vi "Lock Topic.vi"(6 "PublicationPolicy":refnum<class "IPublicationPolicy.lvclass">, 8 "error in (no error)":errorcluster, 9 "Return Error Transport":refnum<class "ITransport.lvclass">, 10 "Publisher ID":string, 11 "Topic in":refnum<class "Topic.lvclass">) -> (0 "error out":errorcluster, 3 "Topic out":refnum<class "Topic.lvclass">)   [LabVIEW 2017, in "Mediator.lvlib" / "Topic.lvclass"]
doc: "<License>\nCopyright © 2017 Composed Systems, LLC | All rights reserved\nwww.composed.io\n\nAuthor: Ethan Stern <ethan.stern@composed.io>\n\nThis software is provided \"AS IS\" WITHOUT WARRANTIES, either express or implied, AND IS FOR EDUCATIONAL PURPOSES ONLY.\n</License>"
uses:
  <vilib>/gpm_packages/@cs/mva-core/Source/Mediator/Topic/Topic.lvclass
  <vilib>/gpm_packages/@cs/transport/Source/ITransport/ITransport.lvclass
  <vilib>/gpm_packages/@cs/mva-core/Source/IMediator/IPublicationPolicy/IPublicationPolicy.lvclass
  <vilib>/gpm_packages/@cs/mva-core/Source/Mediator/Topic/Topic.lvclass/Topic.ctl
  <vilib>/ErrorRing/Error Ring.xnode
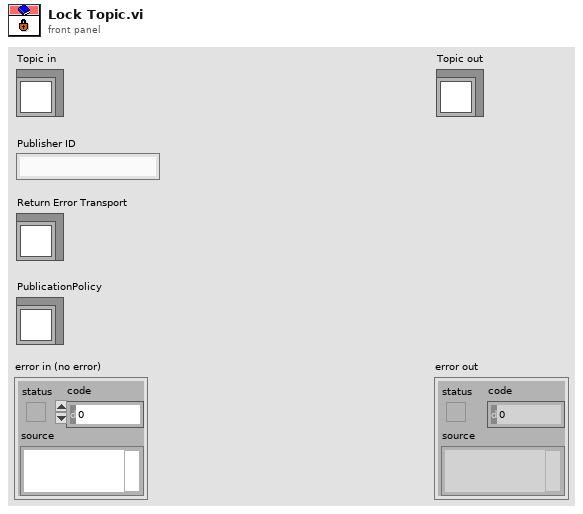
[diagram p1: front panel]
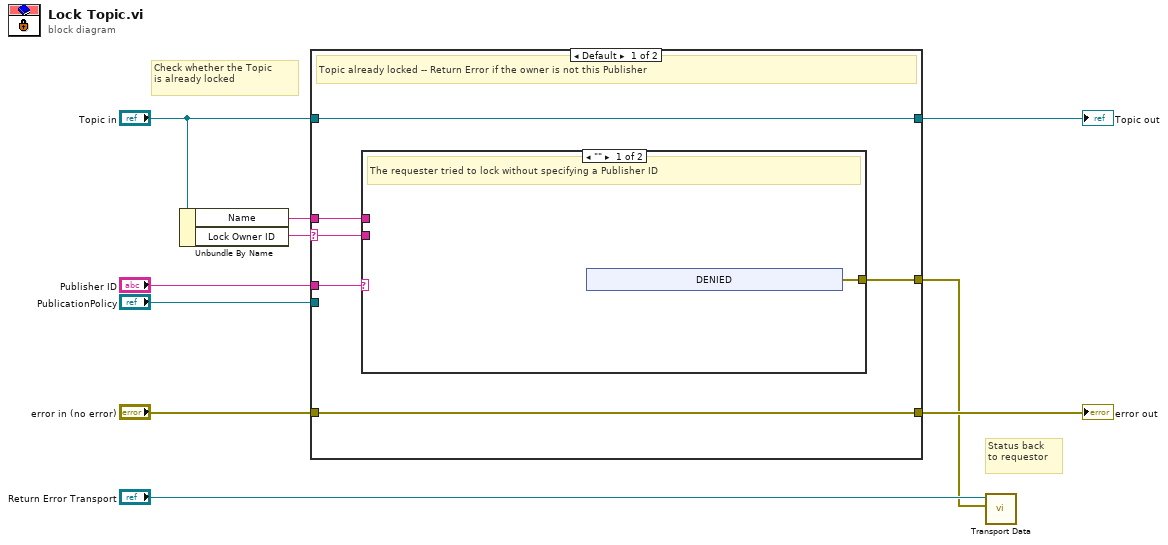
[diagram p0: block diagram]
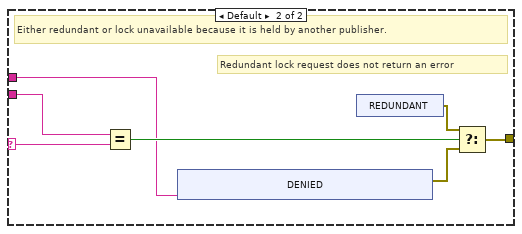
[diagram p2: hidden frame]
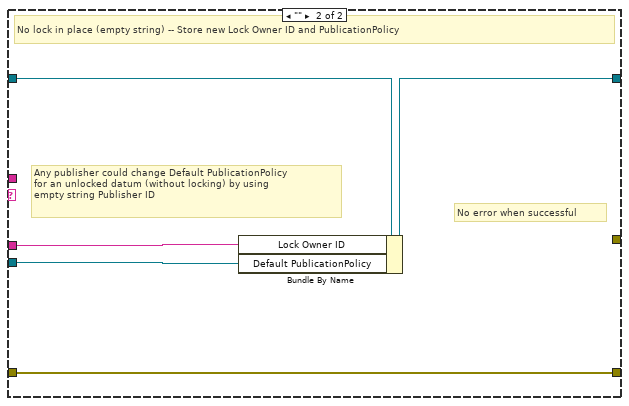
[diagram p3: hidden frame]
diagram:
  # "Status back\nto requestor"
  # "Check whether the Topic\nis already locked"
  n1 = Unbundle By Name("Topic in") -> ("Name"=w1:string, "Lock Owner ID"=w4:string)
  n2 = case shown="Default" w4 {
    selector: w4 -> [w15 _]
    tunnel: "error in (no error)" -> [w16 w33]
    tunnel: [w16 w33] -> w9
    tunnel: [w13 w35] -> w8
    tunnel: "Topic in" -> [w13 w36]
    tunnel: "Publisher ID" -> [w14 w34]
    tunnel: "PublicationPolicy" -> [_ w32]
    tunnel: [w12 _] -> w2
    tunnel: w1 -> [w11 _]
    frame Default {
      # "Topic already locked -- Return Error if the owner is not this Publisher"
      n3 = case shown="\"\"" w14 {
        selector: w14 -> [_ w24]
        tunnel: w15 -> [_ w25]
        tunnel: [w17 w20] -> w12
        tunnel: w11 -> [_ w19]
        frame "" {
          # "The requester tried to lock without specifying a Publisher ID"
          n4 = xnode "DENIED"() -> ("error out"=w17:errorcluster)
        }
        frame Default {
          # "Redundant lock request does not return an error"
          # "Either redundant or lock unavailable because it is held by another publisher."
          n5 = Equal?(x=w25, y=w24) -> (x = y?=w23:bool)
          n6 = xnode "DENIED"("parameter 0"=w19) -> ("error out"=w21:errorcluster)
          n7 = xnode "REDUNDANT"() -> ("error out"=w22:errorcluster)
          n8 = Select(t=w22, s=w23, f=w21) -> (s? t:f=w20:errorcluster)
        }
      }
    }
    frame "" {
      # "No error when successful"
      # "Any publisher could change Default PublicationPolicy\nfor an unlocked datum (without locking) by using\nempty string Publisher ID"
      # "No lock in place (empty string) -- Store new Lock Owner ID and PublicationPolicy"
      n9 = Bundle By Name(cluster=w36, "Lock Owner ID"=w34, "Default PublicationPolicy"=w32) -> (w35:refnum<class "Topic.lvclass">)
    }
  }
  "error out" <- w9
  "Topic out" <- w8
  n10 = call <vilib>:"Transport Data.vi"("Value"=w2, "ITransport in"="Return Error Transport") -> ()  [unwired: 8 in, 2 out]
